vi "Read data HW.vi"(8 "error in":errorcluster, 11 "HW Resource in":T1) -> (0 "error out":errorcluster, 2 "data":waveform(dbl)[](array[waveform]), 3 "HW Resource out":T1)   [LabVIEW 2017]
uses:
  Control/Config chanel.ctl
  <vilib>/DAQmx/read.llb/DAQmx Read (Analog 1D Wfm NChan NSamp).vi
  <vilib>/DAQmx/miscellaneous.llb/DAQmx Fill In Error Info.vi
  <resource>/objmgr/daqmx.rc
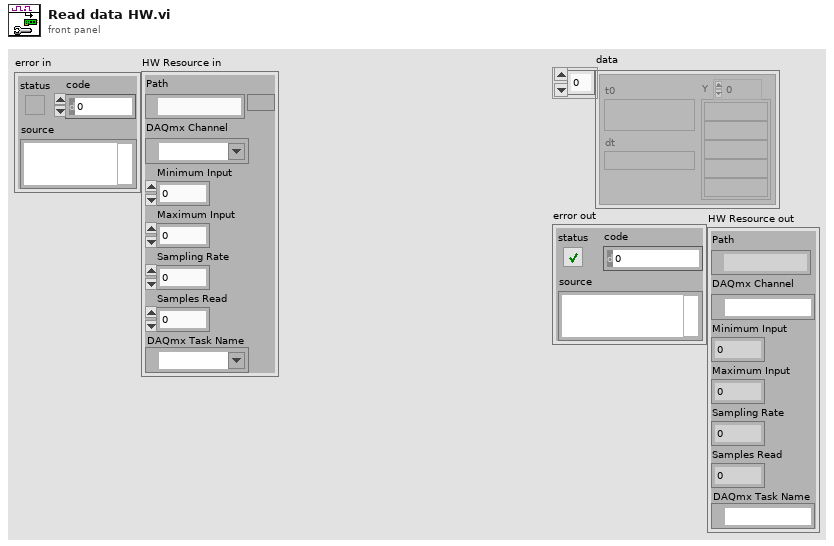
[diagram p1: front panel]
types:
  T1 = typedef "Config chanel.ctl" = cluster{"Path":path, "DAQmx Channel":tag, "Minimum Input":dbl, "Maximum Input":dbl, "Sampling Rate":dbl, "Samples Read":dbl, "DAQmx Task Name":refnum<k21>}
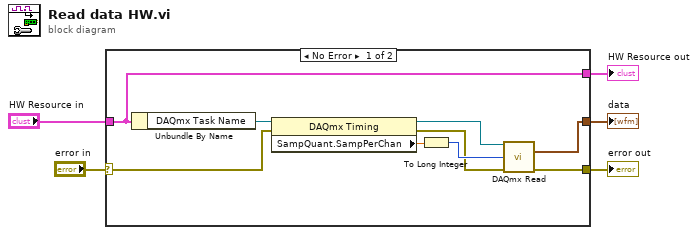
[diagram p0: block diagram]
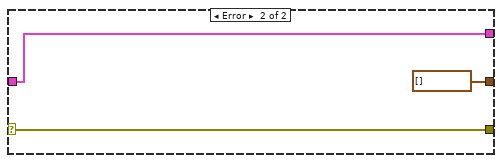
[diagram p2: hidden frame]
diagram:
  n1 = case shown="No Error" "error in" {
    selector: "error in" -> [w7 w17]
    tunnel: "HW Resource in" -> [w11 w15]
    tunnel: [w14 waveform(dbl)[] [] ("data")] -> w4
    tunnel: [w13 w17] -> w2
    tunnel: [w11 w15] -> w1
    frame No Error {
      n2 = Unbundle By Name(w11) -> ("DAQmx Task Name"=w10:refnum<k21>)
      n3 = property class="DAQmx Timing"(reference=w10, error in=w7) -> (reference out=w9:refnum<k21>, error out=w6:errorcluster, "SampQuant.SampPerChan"=w8:dbl)
      n4 = To Long Integer(number=w8) -> (32bit integer=w12:i32)
      n5 = call-poly <vilib>:"DAQmx Read.vi"("task/channels in"=w9, "number of samples per channel"=w12, "error in"=w6) -> ("data"=w14:waveform(dbl)[], "error out"=w13:errorcluster)  [unwired: 10 in, 1 out]
    }
    frame Error {
    }
  }
  "data" <- w4
  "error out" <- w2
  "HW Resource out" <- w1
